vi "Delete.vi"(8 "error in (no error)":errorcluster, 11 "Virtual Memory Unit in":refnum<class "Virtual Memory Unit.lvclass">) -> (0 "error out":errorcluster)   [LabVIEW 2020, in "BCI-1553 API.lvlib" / "Virtual Memory.lvlib" / "Virtual Memory Unit.lvclass"]
doc: "Destroys the Virtual Memory irreversably and releases all the memory allocated by it."
uses:
  Virtual Memory Unit.lvclass
  Virtual Memory Unit.lvclass/Virtual Memory Unit.ctl
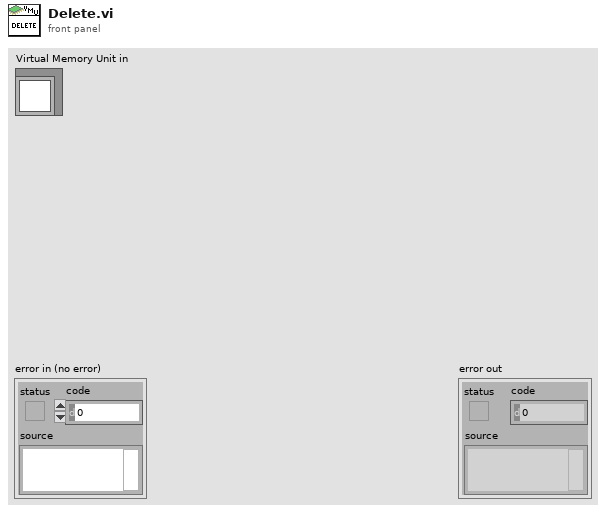
[diagram p1: front panel]
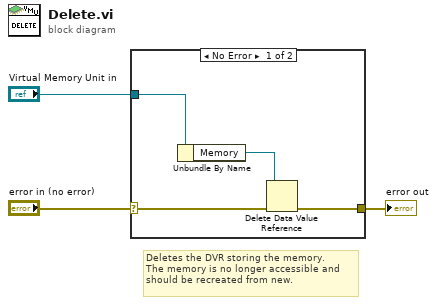
[diagram p0: block diagram]
diagram:
  # "Deletes the DVR storing the memory.\nThe memory is no longer accessible and\nshould be recreated from new."
  n1 = case shown="No Error" "error in (no error)" {
    selector: "error in (no error)" -> [w5 w8]
    tunnel: [w4 w8] -> w2
    tunnel: "Virtual Memory Unit in" -> [w7 _]
    frame No Error {
      n2 = Unbundle By Name(w7) -> ("Memory"=w6:refnum<data-value>)
      n3 = Delete Data Value Reference(data value reference=w6, error in=w5) -> (error out=w4:errorcluster)  [unwired: 1 out]
    }
    frame Error {
    }
  }
  "error out" <- w2
